vi "VI Main 1.21 - Copy.vi"() -> ()   [LabVIEW 2014]
uses:
  <vilib>/Analysis/baseanly.llb/Mean (DBL).vi
  <vilib>/Instr/_visa.llb/VISA Configure Serial Port (Instr).vi
  <vilib>/DAQmx/create/channels.llb/DAQmx Create Channel (AI-Voltage-Basic).vi
  <vilib>/DAQmx/configure/timing.llb/DAQmx Timing (Sample Clock).vi
  <vilib>/DAQmx/read.llb/DAQmx Read (Analog 2D DBL NChan NSamp).vi
  <vilib>/Utility/file.llb/Write To Spreadsheet File (DBL).vi
  <vilib>/Analysis/NI_AALPro.lvlib
  <vilib>/Analysis/NI_AALBase.lvlib
panel:
  out "T  (ºC)":dbl format="%.2g"
  out "RH  (%)":dbl format="%.2g"
  out "Ethanol (%)":dbl format="%.3g"
  out "MFC error IO":errorcluster={"status"=TRUE, "code"=0, "source"="VISA Read in MFC_Setpoint.vi->VI Main 1.21.vi"}
  out "KEITHLEY error IO":errorcluster={"status"=TRUE, "code"=0, "source"="Ke24xx Initialize.vi<ERR>Driver Status:  (Hex 0xBFFF0011) Insufficient location information or the device or resource is not present in the system."}
  out "DAQ error IO":errorcluster={"status"=TRUE, "code"=0, "source"="DAQmx Create Channel (AI-Voltage-Basic).vi:1780002<append>\n<B>Device Specified: </B>Dev2\n\n<B>Task Name: </B>_unnamedTask<29>"}
  out "Array 2":T1(array[cluster])=[{"ID"="-", "P(PSI)"=0.0, "T ºC"=0.0, "MassFlow"=0.0, "Setpoint"=0.0, "Gas"="-\r"}] {"Setpoint" format="%.2f"; "MassFlow" format="%.2f"}
  out "Linear?":bool=TRUE
  in  "Tab Control":enum32{"CONFIG", "Experiment"}(tab)=enum."Experiment"
  in  "resource RS232":string="ASRL4::INSTR"
  in  "resource GPIB":string="GPIB0::24::INSTR"
  out "status":i32=-1073807343 format="%.0x"
  in  "Reset":bool
  in  "COM:":bool=TRUE
  in  "RH/T Sensor VSS (V)":dbl=5.05 format="%.3g"
  in  "DAQ channels":tag="Dev1/ai21:23"
  in  "Rate (Hz)":dbl=1000.0
  in  "samples/channel":i32=100
  in  "K0":dbl=0.9054 format="%#_13g"
  in  "K1":dbl=-2.995 format="%#_13g"
  in  "Offset":dbl step=0.01 format="%_3f"
  in  "Gain":dbl=1.0
  in  "VISA COM Port":refnum<visa-resource-name>="COM3"
  in  "baud rate (9600)":u32=19200
  in  "Device ID's":string[](array[string])=["A", "B"]
  in  "Tare Flow":bool
  in  "Tare absP":bool
  in  "Disable MFC":bool
  in  "set 2":bool
  in  "MFC set2":cluster{"String":string, "MFC set":dbl}[](array[cluster])=[{"String"="A", "MFC set"=900.0}, {"String"="B", "MFC set"=100.0}] {"MFC set" format="%.2f"}
  in  "Speed":i32(slide)=2
  in  "# of points to acquire":i32=50 min=1 max=2500 step=1
  in  "Start (V)":dbl step=1.0 format="%.4p"
  in  "Ranging":i32(slide)
  in  "Direction":i32(slide)
  in  "Source compliance (A)":dbl=0.01 format="%.4f"
  in  "Stop (V)":dbl=5.0 format="%.4f"
  in  "Sense range":i32(slide)
  in  "Interval (s)":dbl=1.0 min=1.0 step=1.0
  in  "# of Intervals":i32=60 min=2 step=1
  out "Benchmark (s)":dbl format="%.2g"
  out "Current Interval":i32
  in  "Linear Fit \nResidue Threshold":dbl=0.1 format="%.3g"
  in  "clear graph":bool
  in  "clear graph at start":bool=TRUE
  in  "set 1":bool
  out "None linear \nIntervals":dbl[](array[numeric])
  in  "MFC set1":cluster{"String":string, "MFC set":dbl}[](array[cluster])=[{"String"="A", "MFC set"=1000.0}, {"String"="B", "MFC set"=100.0}] {"MFC set" format="%.2f"}
  in  "IV file path":path
  in  "Save IV to File":bool
  out "Start time":timestamp=timestamp(3638365108.305079 s since 1904-01-01)
  out "Elapsed Time":dbl format="%<%H:%M:%S>t"
  out "residue":dbl format="%#_3g"
  out "Measuring!":bool
  in  "STOP acq":bool
  in  "Quick Acq":bool
  in  "Multi Acq":bool
  in  "Single Acq":bool
  in  "stop":bool
  out "intercept":dbl format="%_4g"
  out "Waveform Chart":T2(graph)={"residue"=0.0, "residue"=0.0, "residue"=0.0, "residue"=0.0, "residue"=883.5, "residue"=0.0}
  out "Res. (ohm)":dbl format="%#.5g"
  out "XY Graph":cluster{dbl[], "Best Linear Fit":dbl[]}[](graph)
  out "Qrun":bool
  out "Mrun":bool
  out "Srun":bool
  # "Ethanol Sensor"
  # "RH%/T Sensor"
  # "MFC's"
  # "KEITHLEY"
  # ">"
  # "by L.Andrzejewski\nlandrzej@uottawa.ca"
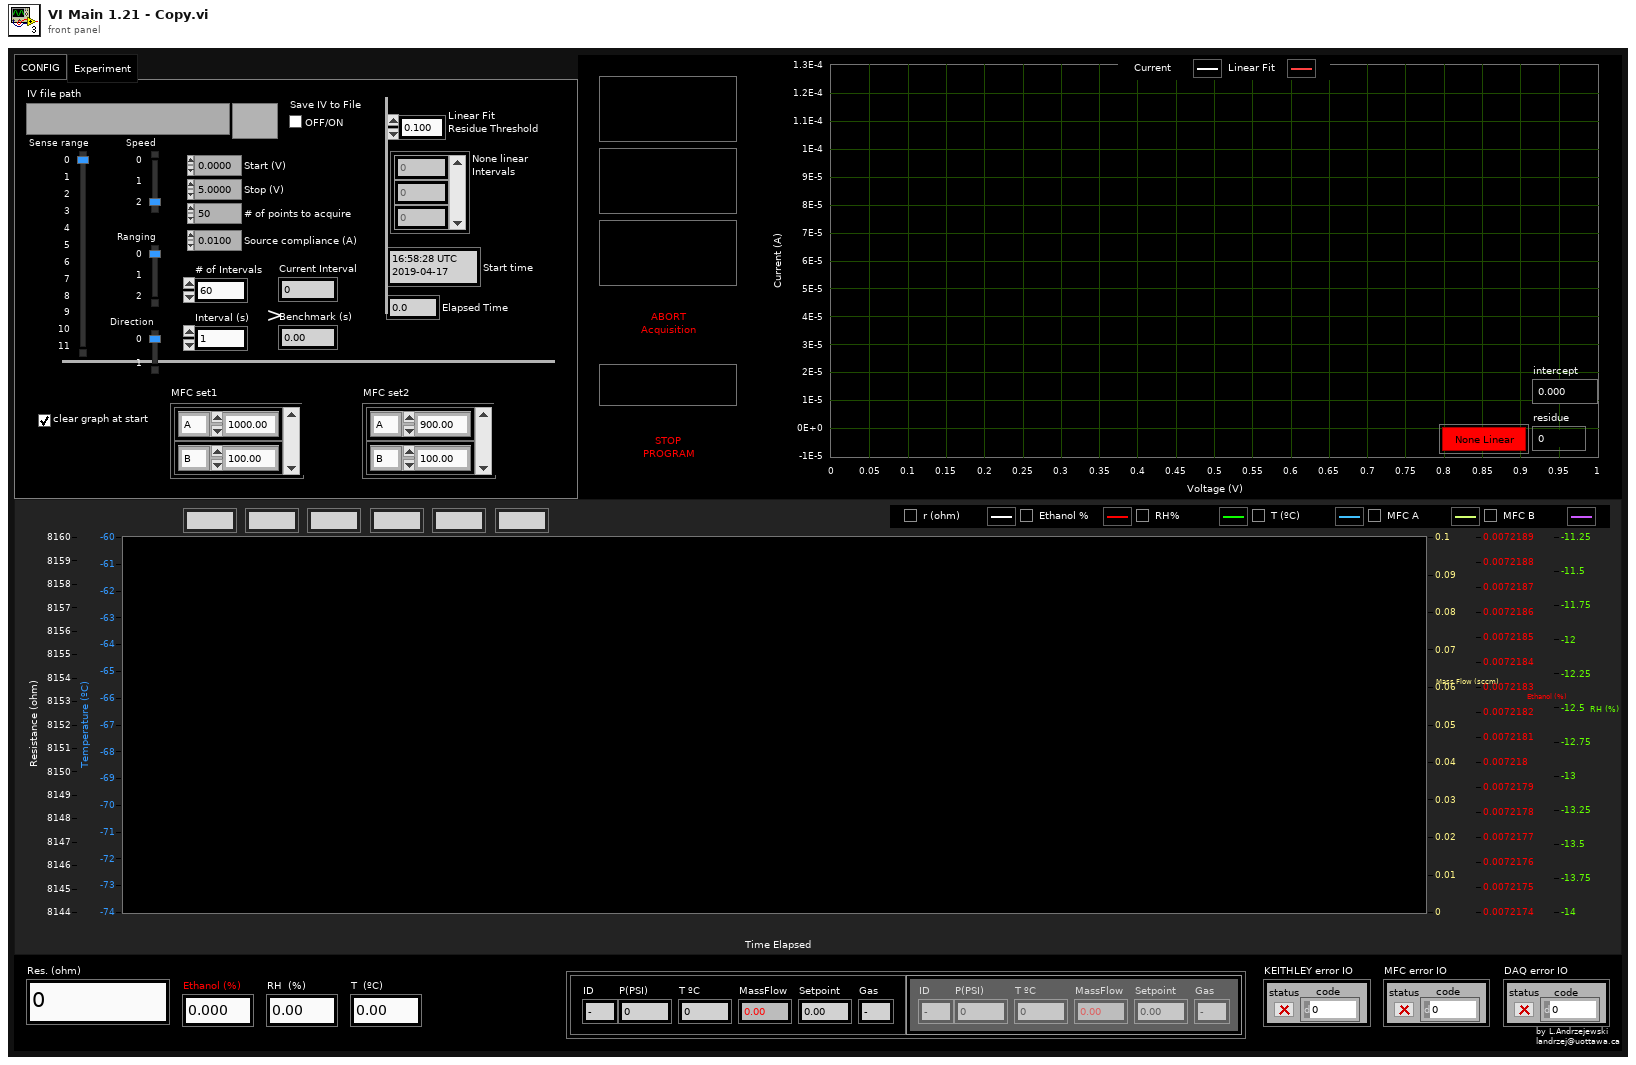
[diagram p1: front panel]
types:
  T1 = cluster{"ID":string, "P(PSI)":dbl, "T ºC":dbl, "MassFlow":dbl, "Setpoint":dbl, "Gas":string}[]
  T2 = cluster{"residue":dbl, "residue":dbl, "residue":dbl, "residue":dbl, "residue":dbl, "residue":dbl}
  T3 = enum8{"Enabled", "Disabled", "Disabled and Grayed Out"}
  T4 = cluster{"residue":dbl, "residue":dbl, "residue":dbl, "residue":dbl, "residue":dbl, "residue":dbl}[]
  T5 = cluster{dbl, dbl, dbl, dbl, "residue":dbl, "residue":dbl}
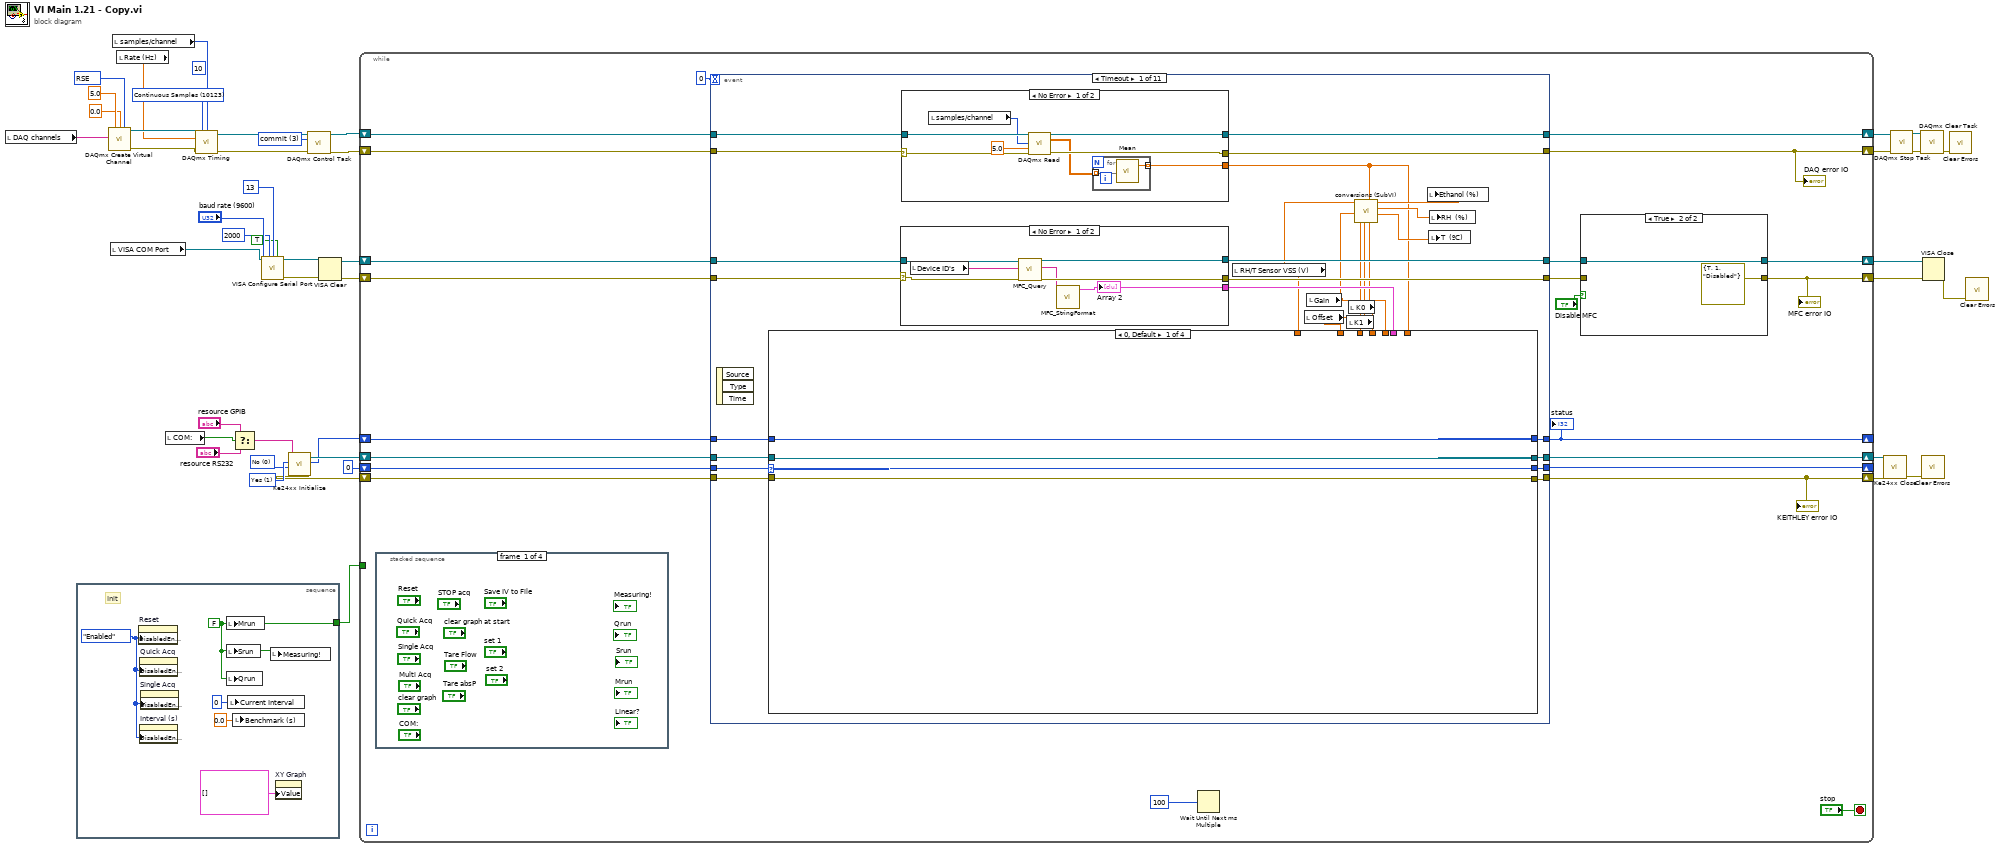
[diagram p0: block diagram]
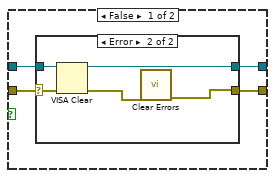
[diagram p2: hidden frame]
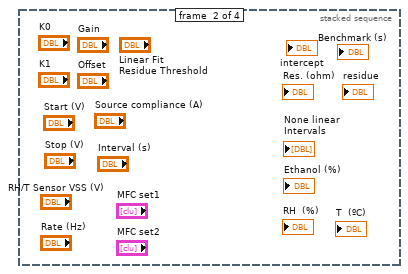
[diagram p4: hidden frame]
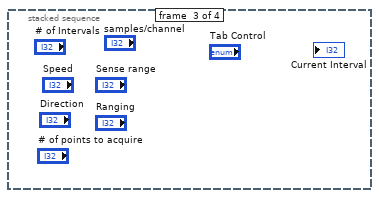
[diagram p5: hidden frame]
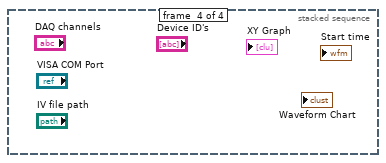
[diagram p6: hidden frame]
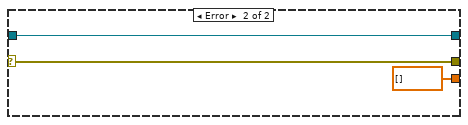
[diagram p7: hidden frame]
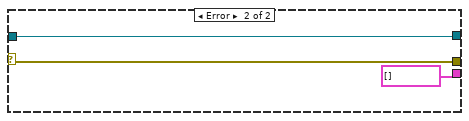
[diagram p8: hidden frame]
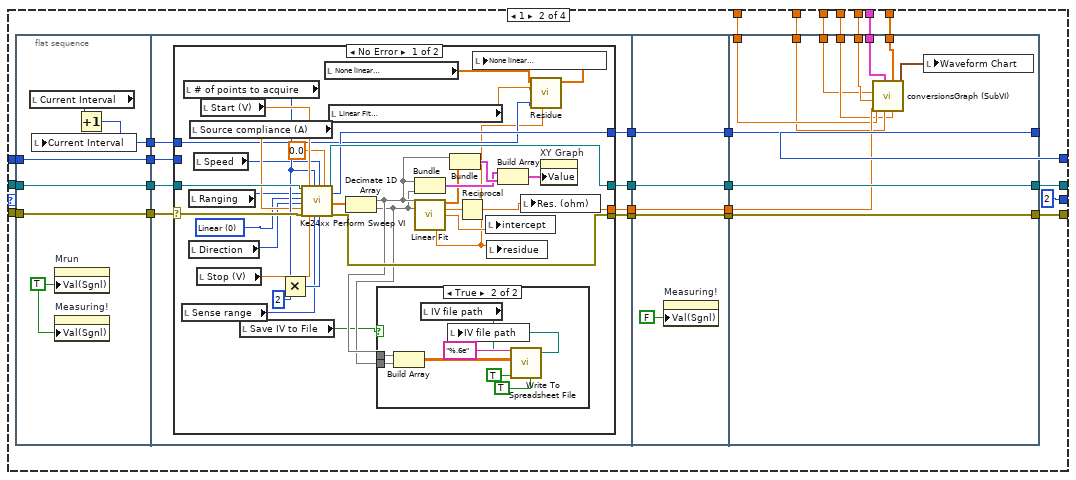
[diagram p9: hidden frame]
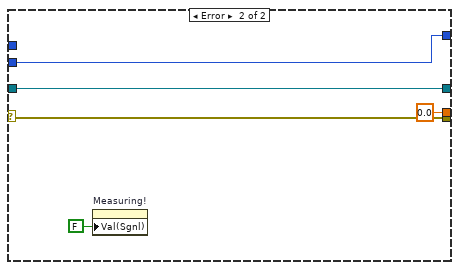
[diagram p11: hidden frame]
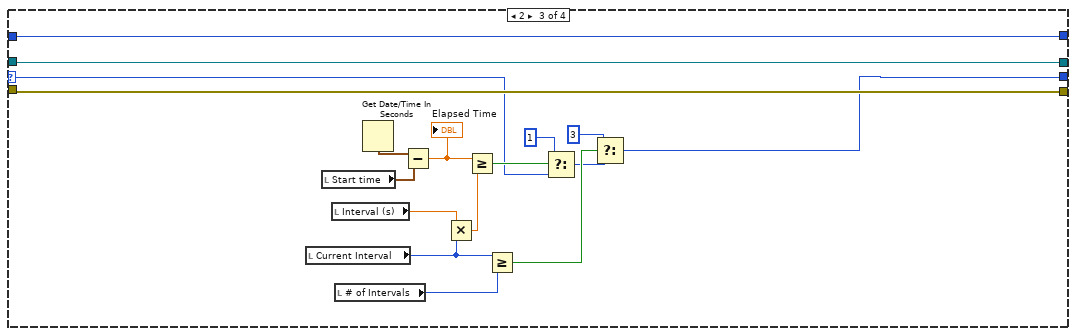
[diagram p12: hidden frame]
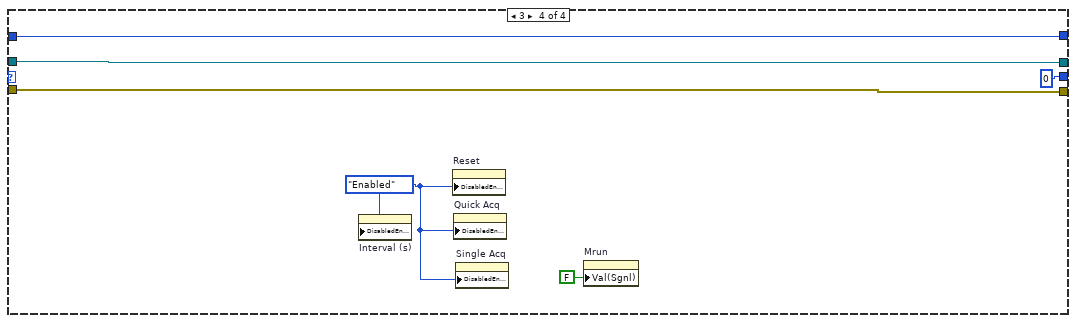
[diagram p13: hidden frame]
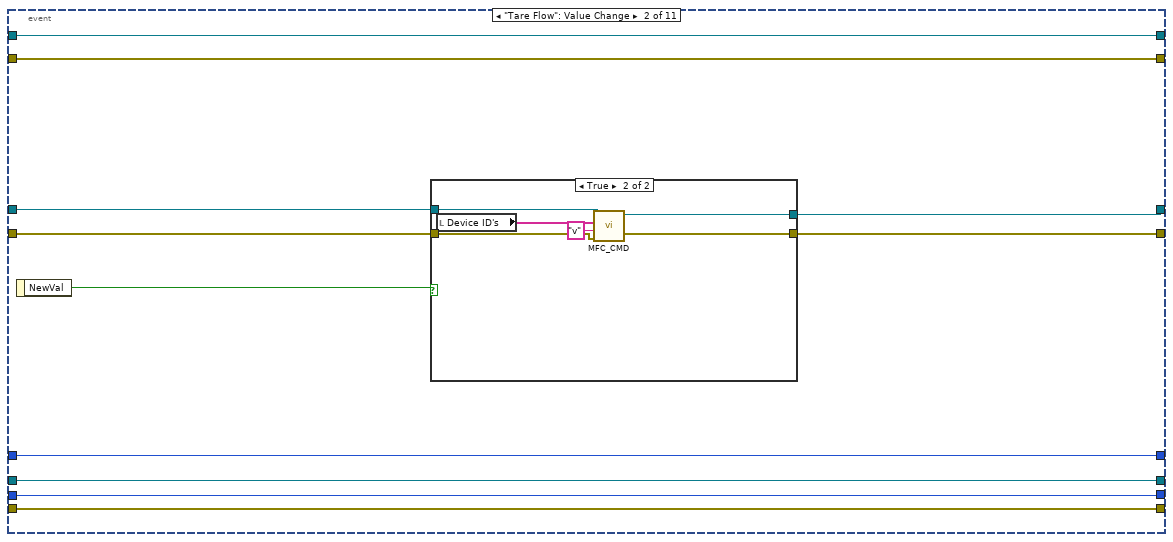
[diagram p14: hidden frame]
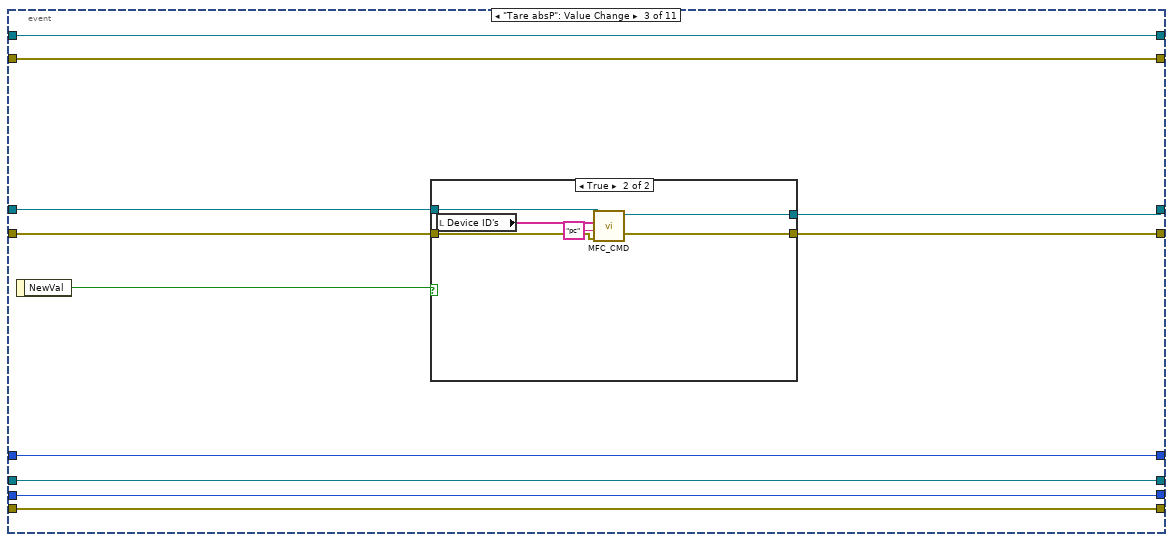
[diagram p16: hidden frame]
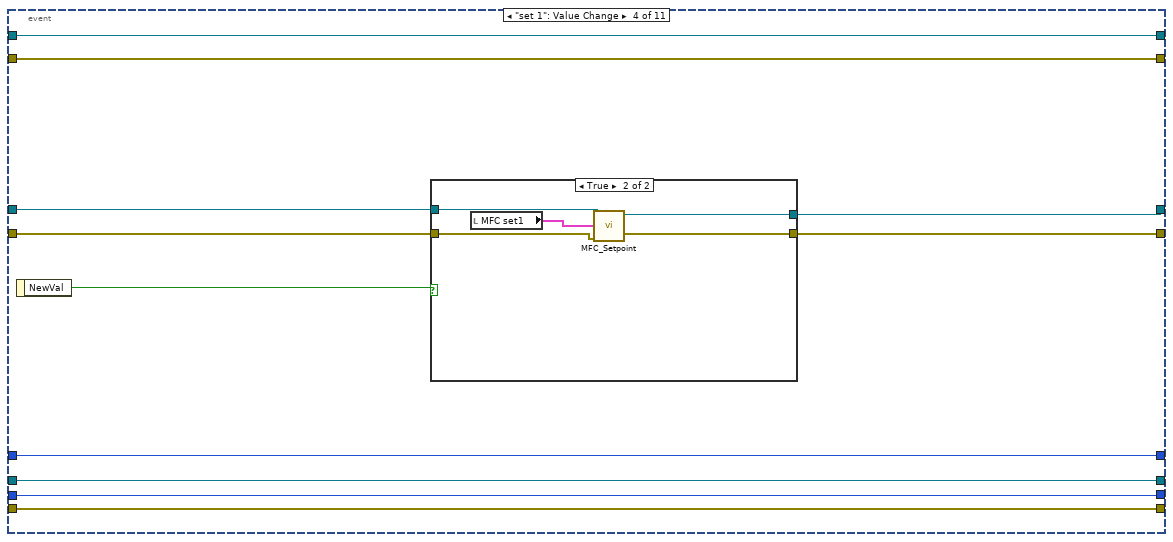
[diagram p18: hidden frame]
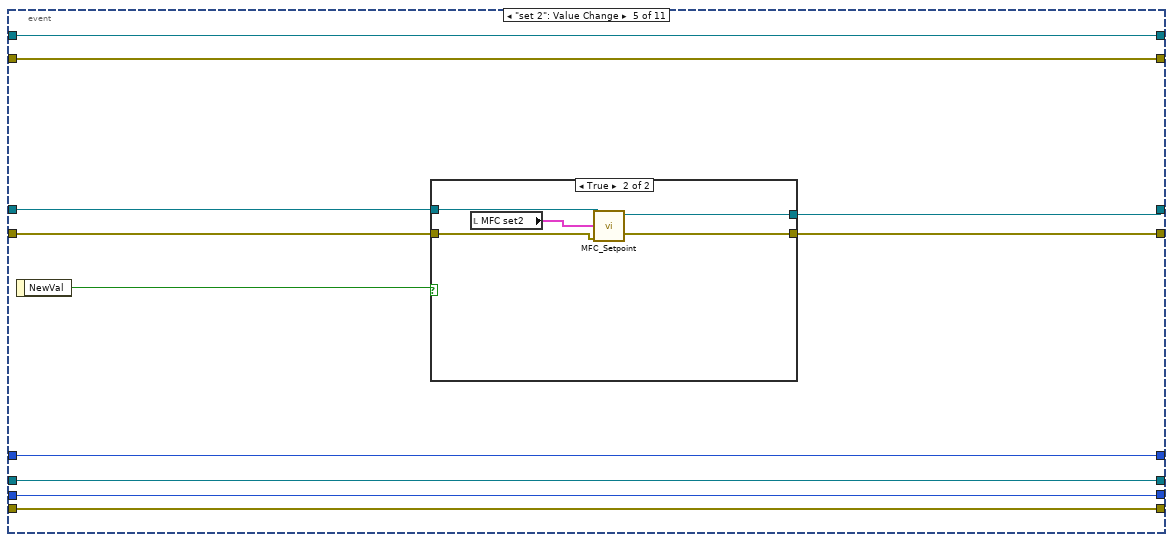
[diagram p20: hidden frame]
diagram:
  (unwired) 10 ("y")
  w3 = 3 items=["verify"=2, "reserve"=4, "commit"=3, "unreserve"=5, "abort"=6] ("action")
  w15 = 10123 items=["Finite Samples"=10178, "Continuous Samples"=10123, "Hardware Timed Single Point"=12522] ("sample mode")
  w17 = 10083 items=["default"=-1, "RSE"=10083, "NRSE"=10078, "Differential"=10106, "Pseudodifferential"=12529] ("input terminal configuration")
  w45 = u16 1 items=["Yes"=1, "No"=0] ("id query")
  w37 = u16 0 items=["Yes"=1, "No"=0] ("reset device")
  n1 = local read "DAQ channels"() -> (w12:tag)
  n2 = stacked-sequence {
    tunnel: [w48] -> w39
    frame #0 {
      w47 = T3."Enabled" ("Disabled")
      w48 = FALSE ("Mrun")
      # "Init"
      n3 = property on="Reset" class="Bool"("DisabledEnum"=w47) -> ()  [unwired: 2 in, 2 out]
      n4 = property on="Quick Acq" class="Bool"("DisabledEnum"=w47) -> ()  [unwired: 2 in, 2 out]
      n5 = property on="Interval (s)" class="DigNum (strict)"("DisabledEnum"=w47) -> ()  [unwired: 2 in, 2 out]
      n6 = property on="Single Acq" class="Bool"("DisabledEnum"=w47) -> ()  [unwired: 2 in, 2 out]
      n7 = local write "Mrun"(w48) -> ()
      n8 = local write "Srun"(w48) -> ()
      n9 = local write "Qrun"(w48) -> ()
      n10 = local write "Current Interval"(0 ("Current Interval")) -> ()
      n11 = local write "Benchmark (s)"(0.0 ("Benchmark (s)")) -> ()
      n12 = local write "Measuring!"(w48) -> ()
      n13 = property on="XY Graph" class="XYGraph (strict)"("Value"=cluster{dbl[], "Best Linear Fit":dbl[]}[] [] ("XY Graph")) -> ()  [unwired: 2 in, 2 out]
    }
  }
  n14 = call-poly <vilib>:"DAQmx Create Virtual Channel.vi"("maximum value"=5.0, "minimum value"=0.0, "input terminal configuration"=w17, "physical channels"=w12) -> ("task out"=w16:refnum<k21>, "error out"=w14:errorcluster)  [unwired: 10 in]
  n15 = local read "VISA COM Port"() -> (w20:refnum<visa-resource-name>)
  n16 = local read "samples/channel"() -> (w2:i32)
  n17 = local read "Rate (Hz)"() -> (w13:dbl)
  n18 = local read "COM:"() -> (w36:bool)
  n19 = call-poly <vilib>:"DAQmx Timing.vi"("task/channels in"=w16, "sample mode"=w15, "samples per channel"=w2, "rate"=w13, "error in"=w14) -> ("task out"=w1:refnum<k21>, "error out"=w4:errorcluster)  [unwired: 9 in]
  n20 = Select(t="resource GPIB", s=w36, f="resource RS232") -> (s? t:f=w33:string)
  n21 = call-poly "VISA Configure Serial Port"("VISA resource name"=w20, "timeout (10sec)"=u32 2000, "termination char\n(0xA = '\\n' = LF)"=u8 13 ("termination char\n(0xA = '\\n' = LF)"), "Enable Termination\nChar (T)"=TRUE ("Enable Termination\nChar (T)"), "baud rate (9600)"="baud rate (9600)") -> ("VISA resource name out"=w22:refnum<visa-resource-name>, "error out"=w21:errorcluster)  [unwired: 9 in]
  n22 = call "Ke24xx Initialize.vi"("reset device"=w37, "id query"=w45, "resource name"=w33) -> ("error out"=w40:errorcluster, "status"=w41:i32, "instrument handle out"=w42:refnum<visa-resource-name>)  [unwired: 6 in]
  n23 = call <vilib>:"DAQmx Control Task.vi"("task/channels in"=w1, "action"=w3, "error in"=w4) -> ("task out"=w6:refnum<k21>, "error out"=w5:errorcluster)  [unwired: 11 in]
  n24 = VISA Clear(VISA resource name=w22, error in (no error)=w21) -> (VISA resource name out=w24:refnum<visa-resource-name>, error out=w23:errorcluster)
  n25 = while {
    shift-right: [w67] -> w44
    shift-left: w42 -> [w69]
    shift-right: [w60] -> w43
    shift-left: w40 -> [w68]
    shift-right: [w65] -> _
    shift-left: w41 -> [w66]
    tunnel: w39 -> [_]
    shift-right: [w63] -> _
    shift-left: 0 -> [w64]
    shift-right: [w53] -> w28
    shift-left: w24 -> [w62]
    shift-right: [w55] -> w27
    shift-left: w23 -> [w61]
    shift-right: [w57] -> w9
    shift-left: w6 -> [w59]
    shift-right: [w52] -> w8
    shift-left: w5 -> [w58]
    stop <- "stop" stop-if-true
    n26 = stacked-sequence {
      frame #0 {
      }
      frame #1 {
      }
      frame #2 {
      }
      frame #3 {
      }
    }
    n27 = event shown="[0] Timeout" {
      selector: _ -> [_ _ _ _ _ _ _ _ _ _ _]
      dyn-events: _ -> [_ _ _ _ _ _ _ _ _ _ _]
      timeout: 0 -> [_ _ _ _ _ _ _ _ _ _ _]
      tunnel: [w107 w275 w294 w313 w331 w351 w376 w387 w462 w518 w537] -> w67
      tunnel: w69 -> [w110 w275 w294 w313 w331 w351 w376 w390 w465 w519 w537]
      tunnel: [w106 w273 w292 w311 w329 w350 w375 w388 w463 w517 w535] -> w60
      tunnel: w68 -> [w109 w273 w292 w311 w329 w350 w375 w389 w464 w516 w535]
      tunnel: w66 -> [w108 w272 w291 w310 w328 w347 w372 w386 w461 w521 w538]
      tunnel: [w104 w272 w291 w310 w328 w347 w372 w385 w460 w520 w538] -> w65
      tunnel: w64 -> [w111 w274 w293 w312 w330 w348 w373 w384 w459 w515 w536]
      tunnel: [w105 w274 w293 w312 w330 w349 w374 w384 w459 w515 w536] -> w63
      tunnel: [w102 w268 w287 w306 w324 w345 w370 w382 w457 w513 w533] -> w54
      tunnel: w62 -> [w97 w270 w289 w308 w326 w345 w370 w382 w457 w513 w533]
      tunnel: [w103 w267 w286 w305 w323 w346 w371 w383 w458 w514 w534] -> w56
      tunnel: w61 -> [w96 w269 w288 w307 w325 w346 w371 w383 w458 w514 w534]
      tunnel: [w99 w266 w285 w304 w322 w344 w369 w381 w456 w512 w532] -> w57
      tunnel: w59 -> [w86 w266 w285 w304 w322 w344 w369 w381 w456 w512 w532]
      tunnel: [w98 w265 w284 w303 w321 w343 w368 w380 w455 w511 w531] -> w52
      tunnel: w58 -> [w100 w265 w284 w303 w321 w343 w368 w380 w455 w511 w531]
      event Timeout {
        n28 = event-data() -> ()  [unwired: 1 in, 3 out]
        n29 = case shown="No Error" w96 {
          selector: w96 -> [w129 w133]
          tunnel: w97 -> [w130 w134]
          tunnel: [w128 w133] -> w103
          tunnel: [w127 w134] -> w102
          tunnel: [w125 T1 [] ("Array out")] -> w101
          frame No Error {
            n30 = local read "Device ID's"() -> (w131:string[])
            n31 = call "MFC_Query.vi"("error in (no error)"=w129, "Device ID's"=w131, "VISA Refnum in"=w130) -> ("error out"=w128:errorcluster, "Array"=w126:string[], "VISA Refnum out"=w127:refnum<visa-resource-name>)  [unwired: 6 in]
            n32 = call "MFC_StringFormat.vi"("Array"=w126) -> ("Array out"=w125:T1)  [unwired: 10 in]
            "Array 2" <- w125
          }
          frame Error {
          }
        }
        n33 = case shown="No Error" w100 {
          selector: w100 -> [w115 w123]
          tunnel: [w118 w124] -> w99
          tunnel: w86 -> [w119 w124]
          tunnel: [w114 w123] -> w98
          tunnel: [w112 dbl[] []] -> w92
          frame No Error {
            n34 = local read "samples/channel"() -> (w116:i32)
            n35 = call-poly <vilib>:"DAQmx Read.vi"("task/channels in"=w119, "number of samples per channel"=w116, "timeout"=5.0, "error in"=w115) -> ("task out"=w118:refnum<k21>, "data"=w113:dbl[][], "error out"=w114:errorcluster)  [unwired: 9 in]
            n36 = for {
              tunnel: w113 -> [w121] mode=indexing
              tunnel: [w120] -> w112 mode=indexing
              n37 = call-poly <vilib>:"Mean.vi"("X"=w121) -> ("mean"=w120:dbl)  [unwired: 1 out]
            }
          }
          frame Error {
          }
        }
        n38 = local read "RH/T Sensor VSS (V)"() -> (w91:dbl)
        n39 = local read "Offset"() -> (w88:dbl)
        n40 = local read "Gain"() -> (w89:dbl)
        n41 = local read "K1"() -> (w90:dbl)
        n42 = local read "K0"() -> (w87:dbl)
        n43 = case shown="0, Default" w111 {
          selector: w111 -> [w135 _ w247 _]
          tunnel: w110 -> [w137 w162 w256 w262]
          tunnel: w109 -> [w136 w161 w257 w260]
          tunnel: w108 -> [w138 w145 w258 w263]
          tunnel: [w137 w160 w256 w262] -> w107
          tunnel: [w136 w159 w257 w260] -> w106
          tunnel: [w135 2 w244 0 ("t")] -> w105
          tunnel: [w138 w157 w258 w263] -> w104
          tunnel: w101 -> [_ w150 _ _]
          tunnel: w92 -> [_ w149 _ _]
          tunnel: w91 -> [_ w143 _ _]
          tunnel: w89 -> [_ w142 _ _]
          tunnel: w88 -> [_ w141 _ _]
          tunnel: w87 -> [_ w140 _ _]
          tunnel: w90 -> [_ w139 _ _]
          frame 0, Default {
          }
          frame 1 {
            n44 = flat-sequence {
              tunnel: w161 -> [w169]
              tunnel: w162 -> [w170]
              tunnel: [w170] -> w164
              tunnel: [w169] -> w163
              tunnel: [w167] -> w146
              tunnel: w145 -> [w167]
              tunnel: [w165] -> w144
              tunnel: w164 -> [w178]
              tunnel: w163 -> [w177]
              tunnel: [w176] -> w156
              tunnel: [w175] -> w155
              tunnel: [w174] -> w154
              tunnel: [w173] -> w147
              tunnel: w146 -> [w172]
              tunnel: w144 -> [w171]
              tunnel: w156 -> [w229]
              tunnel: w155 -> [w228]
              tunnel: w154 -> [w227]
              tunnel: [w229] -> w153
              tunnel: [w228] -> w152
              tunnel: [w227] -> w151
              tunnel: [w225] -> w148
              tunnel: w147 -> [w225]
              tunnel: [w239] -> w157
              tunnel: [w240] -> w160
              tunnel: [w241] -> w159
              tunnel: w153 -> [w241]
              tunnel: w152 -> [w240]
              tunnel: w151 -> [w239]
              tunnel: w150 -> [w235]
              tunnel: w149 -> [w236]
              tunnel: w148 -> [w237]
              tunnel: w143 -> [w234]
              tunnel: w142 -> [w233]
              tunnel: w141 -> [w232]
              tunnel: w140 -> [w231]
              tunnel: w139 -> [w230]
              frame #0 {
                w166 = TRUE ("Value (Signaling)")
                n45 = local read "Current Interval"() -> (w168:i32)
                n46 = property on="Mrun" class="Bool (strict)"("Val(Sgnl)"=w166) -> ()  [unwired: 2 in, 2 out]
                n47 = property on="Measuring!" class="Bool (strict)"("Val(Sgnl)"=w166) -> ()  [unwired: 2 in, 2 out]
                n48 = Increment(x=w168) -> (x+1=w165:i32)
                n49 = local write "Current Interval"(w165) -> ()
              }
              frame #1 {
                n50 = case shown="No Error" w177 {
                  selector: w177 -> [w205 w223]
                  tunnel: w178 -> [w206 w224]
                  tunnel: [w204 w223] -> w176
                  tunnel: [w203 w224] -> w175
                  tunnel: [w188 w221] -> w174
                  tunnel: [w187 0.0] -> w173
                  tunnel: w172 -> [_ w221]
                  tunnel: w171 -> [w181 _]
                  frame No Error {
                    w190 = 0 items=["Linear", "Logarithmic"] ("spacing")
                    n51 = local read "Sense range"() -> (w195:i32)
                    n52 = local read "# of points to acquire"() -> (w197:i32)
                    n53 = local read "Ranging"() -> (w192:i32)
                    n54 = local read "Direction"() -> (w191:i32)
                    n55 = local read "Source compliance (A)"() -> (w194:dbl)
                    n56 = local read "Speed"() -> (w193:i32)
                    n57 = local read "Stop (V)"() -> (w199:dbl)
                    n58 = local read "Start (V)"() -> (w200:dbl)
                    n59 = local read "Save IV to File"() -> (w184:bool)
                    n60 = Multiply(x=w197, y=2) -> (x*y=w196:i32)
                    n61 = call "Ke24xx Perform Sweep VI.vi"("instrument handle"=w206, "ranging"=w192, "spacing"=w190, "direction"=w191, "source compliance"=w194, "error in (no error)"=w205, "start"=w200, "stop"=w199, "number of points"=w197, "sense range"=w195, "speed"=w193, "size of reading"=w196, "source protection"=0.0) -> ("instrument handle out"=w203:refnum<visa-resource-name>, "status"=w188:i32, "out"=w207:dbl[], "error out"=w204:errorcluster)  [unwired: 3 in]
                    n62 = local read "None linear \nIntervals"() -> (w183:dbl[])
                    n63 = local read "Linear Fit \nResidue Threshold"() -> (w180:dbl)
                    n64 = Decimate 1D Array(w207) -> (w186:dbl[], w185:dbl[])
                    n65 = case shown="True" w184 {
                      tunnel: w186 -> [_ w219]
                      tunnel: w185 -> [_ w218]
                      frame False {
                      }
                      frame True {
                        n66 = Build Array(w219, w218) -> (w214:dbl[][])
                        n67 = local read "IV file path"() -> (w215:path)
                        n68 = call-poly <vilib>:"Write To Spreadsheet File.vi"("transpose? (no:F)"=TRUE, "format (%.3f)"="%.6e", "append to file? (new file:F)"=TRUE, "2D data"=w214, "file path (dialog if empty)"=w215) -> ("new file path (Not A Path if cancelled)"=w213:path)  [unwired: 3 in]
                        n69 = local write "IV file path"(w213) -> ()
                      }
                    }
                    n70 = Bundle(w186, w185) -> (w210:cluster{dbl[], dbl[]})  [unwired: 1 in]
                    n71 = call <vilib>:"Linear Fit.vi"("Y"=w185, "X"=w186) -> ("Best Linear Fit"=w209:dbl[], "slope"=w208:dbl, "intercept"=w202:dbl, "residue"=w179:dbl)  [unwired: 9 in, 1 out]
                    n72 = Bundle(w186, "Best Linear Fit"=w209) -> (w211:cluster{dbl[], "Best Linear Fit":dbl[]})  [unwired: 1 in]
                    n73 = Reciprocal(x=w208) -> (1/x=w187:dbl)
                    n74 = local write "intercept"(w202) -> ()
                    n75 = local write "residue"(w179) -> ()
                    n76 = Build Array(w210, w211) -> (w201:cluster{dbl[], "Best Linear Fit":dbl[]}[])
                    n77 = local write "Res. (ohm)"(w187) -> ()
                    n78 = call "Residue.vi"("residue"=w179, "Current Interval"=w181, "Linear Fit \nResidue Threshold"=w180, "None linear \nIntervals IN"=w183) -> ("None linear \nIntervals OUT"=w182:dbl[])  [unwired: 7 in]
                    n79 = local write "None linear \nIntervals"(w182) -> ()
                    n80 = property on="XY Graph" class="XYGraph (strict)"("Value"=w201) -> ()  [unwired: 2 in, 2 out]
                  }
                  frame Error {
                    n81 = property on="Measuring!" class="Bool (strict)"("Val(Sgnl)"=FALSE ("Value (Signaling)")) -> ()  [unwired: 2 in, 2 out]
                  }
                }
              }
              frame #2 {
                n82 = property on="Measuring!" class="Bool (strict)"("Val(Sgnl)"=FALSE ("Value (Signaling)")) -> ()  [unwired: 2 in, 2 out]
              }
              frame #3 {
                n83 = call "conversionsGraph (SubVI).vi"("K0"=w231, "Array"=w236, "Offset"=w232, "Array in"=w235, "Numeric"=w237, "Gain"=w233, "K1"=w230, "RH/T Sensor VSS (V)"=w234) -> ("Cluster"=w238:T5)  [unwired: 3 in]
                n84 = local write "Waveform Chart"(w238) -> ()
              }
            }
          }
          frame 2 {
            n85 = local read "Current Interval"() -> (w250:i32)
            n86 = local read "Start time"() -> (w254:timestamp)
            n87 = local read "Interval (s)"() -> (w253:dbl)
            n88 = local read "# of Intervals"() -> (w249:i32)
            n89 = Get Date/Time In Seconds() -> (seconds since 1Jan1904=w255:timestamp)
            n90 = Subtract(x=w255, y=w254) -> (x-y=w242:dbl)
            "Elapsed Time" <- w242
            n91 = Multiply(x=w253, y=w250) -> (x*y=w252:dbl)
            n92 = Greater Or Equal?(x=w242, y=w252) -> (x >= y?=w251:bool)
            n93 = Greater Or Equal?(x=w250, y=w249) -> (x >= y?=w246:bool)
            n94 = Select(t=1, s=w251, f=w247) -> (s? t:f=w245:i32)
            n95 = Select(t=3, s=w246, f=w245) -> (s? t:f=w244:i32)
          }
          frame 3 {
            w259 = T3."Enabled" ("Disabled")
            n96 = property on="Interval (s)" class="DigNum (strict)"("DisabledEnum"=w259) -> ()  [unwired: 2 in, 2 out]
            n97 = property on="Reset" class="Bool"("DisabledEnum"=w259) -> ()  [unwired: 2 in, 2 out]
            n98 = property on="Quick Acq" class="Bool"("DisabledEnum"=w259) -> ()  [unwired: 2 in, 2 out]
            n99 = property on="Single Acq" class="Bool"("DisabledEnum"=w259) -> ()  [unwired: 2 in, 2 out]
            n100 = property on="Mrun" class="Bool (strict)"("Val(Sgnl)"=FALSE ("Value (Signaling)")) -> ()  [unwired: 2 in, 2 out]
          }
        }
        n101 = call "conversions (SubVI).vi"("K0"=w87, "Array"=w92, "Offset"=w88, "Gain"=w89, "K1"=w90, "RH/T Sensor VSS (V)"=w91) -> ("T"=w93:dbl, "RH"=w94:dbl, "Ethanol"=w95:dbl)  [unwired: 3 in]
        n102 = local write "Ethanol (%)"(w95) -> ()
        n103 = local write "T  (ºC)"(w93) -> ()
        n104 = local write "RH  (%)"(w94) -> ()
      }
      event "Tare Flow": Value Change {
        n105 = event-data() -> ("NewVal"=w271:bool)  [unwired: 1 in]
        n106 = case shown="True" w271 {
          tunnel: w270 -> [w277 w283]
          tunnel: w269 -> [w276 w282]
          tunnel: [w277 w281] -> w268
          tunnel: [w276 w280] -> w267
          frame False {
          }
          frame True {
            n107 = local read "Device ID's"() -> (w279:string[])
            n108 = call "MFC_CMD.vi"("error in (no error)"=w282, "cmd"="v", "Device ID's"=w279, "VISA Refnum in"=w283) -> ("error out"=w280:errorcluster, "VISA Refnum out"=w281:refnum<visa-resource-name>)  [unwired: 6 in]
          }
        }
      }
      event "Tare absP": Value Change {
        n109 = event-data() -> ("NewVal"=w290:bool)  [unwired: 1 in]
        n110 = case shown="True" w290 {
          tunnel: w289 -> [w296 w302]
          tunnel: w288 -> [w295 w301]
          tunnel: [w296 w300] -> w287
          tunnel: [w295 w299] -> w286
          frame False {
          }
          frame True {
            n111 = local read "Device ID's"() -> (w298:string[])
            n112 = call "MFC_CMD.vi"("error in (no error)"=w301, "cmd"="pc", "Device ID's"=w298, "VISA Refnum in"=w302) -> ("error out"=w299:errorcluster, "VISA Refnum out"=w300:refnum<visa-resource-name>)  [unwired: 6 in]
          }
        }
      }
      event "set 1": Value Change {
        n113 = event-data() -> ("NewVal"=w309:bool)  [unwired: 1 in]
        n114 = case shown="True" w309 {
          tunnel: w308 -> [w315 w320]
          tunnel: w307 -> [w314 w319]
          tunnel: [w315 w318] -> w306
          tunnel: [w314 w317] -> w305
          frame False {
          }
          frame True {
            n115 = local read "MFC set1"() -> (w316:cluster{"String":string, "MFC set":dbl}[])
            n116 = call "MFC_Setpoint.vi"("error in (no error)"=w319, "MFC set1"=w316, "VISA Refnum in"=w320) -> ("error out"=w317:errorcluster, "VISA Refnum out"=w318:refnum<visa-resource-name>)  [unwired: 7 in]
          }
        }
      }
      event "set 2": Value Change {
        n117 = event-data() -> ("NewVal"=w327:bool)  [unwired: 1 in]
        n118 = case shown="True" w327 {
          tunnel: w326 -> [w333 w338]
          tunnel: w325 -> [w332 w337]
          tunnel: [w333 w336] -> w324
          tunnel: [w332 w335] -> w323
          frame False {
          }
          frame True {
            n119 = local read "MFC set2"() -> (w334:cluster{"String":string, "MFC set":dbl}[])
            n120 = call "MFC_Setpoint.vi"("error in (no error)"=w337, "MFC set1"=w334, "VISA Refnum in"=w338) -> ("error out"=w335:errorcluster, "VISA Refnum out"=w336:refnum<visa-resource-name>)  [unwired: 7 in]
          }
        }
      }
      event "Multi Acq": Value Change {
        n121 = event-data() -> ("NewVal"=w352:bool)  [unwired: 1 in]
        n122 = local read "IV file path"() -> (w339:path)
        n123 = local read "Save IV to File"() -> (w340:bool)
        n124 = Empty String/Path?(string/path=w339) -> (empty?=w342:bool)
        n125 = And(x=w342, y=w340) -> (x .and. y?=w341:bool)
        n126 = case shown="False" w341 {
          tunnel: w352 -> [w355 _]
          tunnel: [w354 0] -> w349
          tunnel: w348 -> [w353 _]
          frame False {
            n127 = case shown="True" w355 {
              tunnel: [w356 1] -> w354
              tunnel: w353 -> [w356 _]
              frame False {
              }
              frame True {
                w360 = T3."Disabled and Grayed Out" ("Disabled")
                n128 = local read "clear graph at start"() -> (w359:bool)
                n129 = Get Date/Time In Seconds() -> (seconds since 1Jan1904=w362:timestamp)
                n130 = local read "Interval (s)"() -> (w361:dbl)
                n131 = local write "Start time"(w362) -> ()
                n132 = property on="Interval (s)" class="DigNum (strict)"("DisabledEnum"=w360) -> ()  [unwired: 2 in, 2 out]
                n133 = local write "Current Interval"(0 ("Current Interval")) -> ()
                n134 = local write "None linear \nIntervals"(dbl[] [] ("None linear Intervals")) -> ()
                n135 = property on="Waveform Chart" class="WFChart (strict)"("XScale.Multiplier"=w361) -> ()  [unwired: 2 in, 2 out]
                n136 = case shown="True" w359 {
                  frame False {
                  }
                  frame True {
                    n137 = property on="Waveform Chart" class="WFChart (strict)"("History Data"=T4 []) -> ()  [unwired: 2 in, 2 out]
                  }
                }
                n138 = property on="Reset" class="Bool"("DisabledEnum"=w360) -> ()  [unwired: 2 in, 2 out]
                n139 = property on="Quick Acq" class="Bool"("DisabledEnum"=w360) -> ()  [unwired: 2 in, 2 out]
                n140 = property on="Single Acq" class="Bool"("DisabledEnum"=w360) -> ()  [unwired: 2 in, 2 out]
                n141 = property on="XY Graph" class="XYGraph (strict)"("Value"=cluster{dbl[], "Best Linear Fit":dbl[]}[] [] ("XY Graph")) -> ()  [unwired: 2 in, 2 out]
              }
            }
          }
          frame True {
            n142 = One Button Dialog(message="File path empty, Multi Acquisition Canceled") -> ()  [unwired: 1 in, 1 out]
          }
        }
      }
      event "STOP acq": Value Change {
        n143 = event-data() -> ("NewVal"=w377:bool)  [unwired: 1 in]
        n144 = case shown="True" w377 {
          tunnel: [w378 3] -> w374
          tunnel: w373 -> [w378 _]
          frame False {
          }
          frame True {
          }
        }
      }
      event "Single Acq": Value Change {
        n145 = event-data() -> ("NewVal"=w391:bool)  [unwired: 1 in]
        n146 = case shown="True" w391 {
          tunnel: w390 -> [w394 w409]
          tunnel: w389 -> [w393 w408]
          tunnel: [w393 w407] -> w388
          tunnel: [w394 w406] -> w387
          tunnel: [w392 w401] -> w385
          tunnel: w386 -> [w392 _]
          frame False {
          }
          frame True {
            n147 = flat-sequence {
              tunnel: w408 -> [w412]
              tunnel: w409 -> [w413]
              tunnel: [w413] -> w403
              tunnel: [w412] -> w402
              tunnel: [w410] -> w398
              tunnel: [w434] -> w405
              tunnel: [w433] -> w404
              tunnel: w403 -> [w436]
              tunnel: w402 -> [w435]
              tunnel: [w417] -> w400
              tunnel: [w453] -> w406
              tunnel: [w454] -> w407
              tunnel: w405 -> [w454]
              tunnel: w404 -> [w453]
              tunnel: [w452] -> w401
              tunnel: w400 -> [w452]
              tunnel: [w450] -> w399
              frame #0 {
                n148 = Tick Count (ms)() -> (millisecond timer value=w410:u32)
                n149 = property on="Srun" class="Bool (strict)"("Val(Sgnl)"=TRUE ("Value (Signaling)")) -> ()  [unwired: 2 in, 2 out]
              }
              frame #1 {
                w419 = 0 items=["Linear", "Logarithmic"] ("spacing")
                n150 = local read "# of points to acquire"() -> (w426:i32)
                n151 = local read "Ranging"() -> (w421:i32)
                n152 = local read "Direction"() -> (w420:i32)
                n153 = local read "Source compliance (A)"() -> (w423:dbl)
                n154 = local read "Speed"() -> (w422:i32)
                n155 = local read "Stop (V)"() -> (w428:dbl)
                n156 = local read "Start (V)"() -> (w429:dbl)
                n157 = local read "Sense range"() -> (w424:i32)
                n158 = local read "Save IV to File"() -> (w416:bool)
                n159 = Multiply(x=w426, y=2) -> (x*y=w425:i32)
                n160 = call "Ke24xx Perform Sweep VI.vi"("instrument handle"=w436, "ranging"=w421, "spacing"=w419, "direction"=w420, "source compliance"=w423, "error in (no error)"=w435, "start"=w429, "stop"=w428, "number of points"=w426, "sense range"=w424, "speed"=w422, "size of reading"=w425, "source protection"=0.0) -> ("instrument handle out"=w433:refnum<visa-resource-name>, "status"=w417:i32, "out"=w437:dbl[], "error out"=w434:errorcluster)  [unwired: 3 in]
                n161 = Decimate 1D Array(w437) -> (w415:dbl[], w414:dbl[])
                n162 = case shown="True" w416 {
                  tunnel: w415 -> [_ w449]
                  tunnel: w414 -> [_ w448]
                  frame False {
                  }
                  frame True {
                    n163 = Build Array(w449, w448) -> (w444:dbl[][])
                    n164 = local read "IV file path"() -> (w445:path)
                    n165 = call-poly <vilib>:"Write To Spreadsheet File.vi"("transpose? (no:F)"=TRUE, "format (%.3f)"="%.6e", "append to file? (new file:F)"=TRUE, "2D data"=w444, "file path (dialog if empty)"=w445) -> ("new file path (Not A Path if cancelled)"=w443:path)  [unwired: 3 in]
                    n166 = local write "IV file path"(w443) -> ()
                  }
                }
                n167 = Bundle(w415, w414) -> (w440:cluster{dbl[], dbl[]})  [unwired: 1 in]
                n168 = call <vilib>:"Linear Fit.vi"("Y"=w414, "X"=w415) -> ("Best Linear Fit"=w439:dbl[], "slope"=w438:dbl, "intercept"=w432:dbl)  [unwired: 9 in, 2 out]
                n169 = Bundle(w415, "Best Linear Fit"=w439) -> (w441:cluster{dbl[], "Best Linear Fit":dbl[]})  [unwired: 1 in]
                n170 = Reciprocal(x=w438) -> (1/x=w431:dbl)
                n171 = local write "intercept"(w432) -> ()
                n172 = Build Array(w440, w441) -> (w430:cluster{dbl[], "Best Linear Fit":dbl[]}[])
                n173 = local write "Res. (ohm)"(w431) -> ()
                n174 = property on="XY Graph" class="XYGraph (strict)"("Value"=w430) -> ()  [unwired: 2 in, 2 out]
              }
              frame #2 {
                n175 = Tick Count (ms)() -> (millisecond timer value=w450:u32)
                n176 = property on="Srun" class="Bool (strict)"("Val(Sgnl)"=FALSE ("Value (Signaling)")) -> ()  [unwired: 2 in, 2 out]
              }
            }
            n177 = Subtract(x=w399, y=w398) -> (x-y=w397:u32)
            n178 = Divide(x=w397, y=u32 1000) -> (x/y=w395:dbl)
            n179 = local write "Benchmark (s)"(w395) -> ()
          }
        }
      }
      event "Quick Acq": Value Change {
        n180 = event-data() -> ("NewVal"=w466:bool)  [unwired: 1 in]
        n181 = case shown="True" w466 {
          tunnel: w465 -> [w469 w479]
          tunnel: w464 -> [w468 w478]
          tunnel: [w468 w477] -> w463
          tunnel: [w469 w476] -> w462
          tunnel: [w467 w471] -> w460
          tunnel: w461 -> [w467 _]
          frame False {
          }
          frame True {
            n182 = flat-sequence {
              tunnel: w478 -> [w481]
              tunnel: w479 -> [w482]
              tunnel: [w482] -> w475
              tunnel: [w481] -> w474
              tunnel: w475 -> [w502]
              tunnel: w474 -> [w501]
              tunnel: [w500] -> w473
              tunnel: [w499] -> w472
              tunnel: [w485] -> w470
              tunnel: [w509] -> w476
              tunnel: [w510] -> w477
              tunnel: w473 -> [w510]
              tunnel: w472 -> [w509]
              tunnel: [w507] -> w471
              tunnel: w470 -> [w507]
              frame #0 {
                n183 = property on="Qrun" class="Bool (strict)"("Val(Sgnl)"=TRUE ("Qrun")) -> ()  [unwired: 2 in, 2 out]
              }
              frame #1 {
                w486 = 2 items=["Slow", "Medium", "Fast"] ("speed")
                w487 = 2 ("x")
                w489 = 0 items=["Linear", "Logarithmic"] ("spacing")
                n184 = local read "Ranging"() -> (w491:i32)
                n185 = local read "Direction"() -> (w490:i32)
                n186 = local read "Source compliance (A)"() -> (w492:dbl)
                n187 = local read "Stop (V)"() -> (w496:dbl)
                n188 = local read "Start (V)"() -> (w497:dbl)
                n189 = local read "Sense range"() -> (w493:i32)
                n190 = Multiply(x=w487, y=2) -> (x*y=w494:i32)
                n191 = call "Ke24xx Perform Sweep VI.vi"("instrument handle"=w502, "ranging"=w491, "spacing"=w489, "direction"=w490, "source compliance"=w492, "error in (no error)"=w501, "start"=w497, "stop"=w496, "number of points"=w487, "sense range"=w493, "speed"=w486, "size of reading"=w494, "source protection"=0.0) -> ("instrument handle out"=w499:refnum<visa-resource-name>, "status"=w485:i32, "out"=w503:dbl[], "error out"=w500:errorcluster)  [unwired: 3 in]
                n192 = Decimate 1D Array(w503) -> (w506:dbl[], w504:dbl[])
                n193 = call <vilib>:"Linear Fit.vi"("Y"=w504, "X"=w506) -> ("slope"=w505:dbl, "intercept"=w498:dbl, "residue"=w483:dbl)  [unwired: 9 in, 2 out]
                n194 = Reciprocal(x=w505) -> (1/x=w484:dbl)
                n195 = local write "intercept"(w498) -> ()
                n196 = local write "residue"(w483) -> ()
                n197 = local write "Res. (ohm)"(w484) -> ()
              }
              frame #2 {
                n198 = property on="Qrun" class="Bool (strict)"("Val(Sgnl)"=FALSE ("Qrun")) -> ()  [unwired: 2 in, 2 out]
              }
            }
          }
        }
      }
      event "Reset": Value Change {
        n199 = event-data() -> ("NewVal"=w522:bool)  [unwired: 1 in]
        n200 = case shown="True" w522 {
          tunnel: [w525 w526] -> w520
          tunnel: w521 -> [w525 _]
          tunnel: w519 -> [w524 w530]
          tunnel: [w524 w529] -> w518
          tunnel: [w523 w527] -> w517
          tunnel: w516 -> [w523 w528]
          frame False {
          }
          frame True {
            n201 = call "Ke24xx Reset.vi"("error in (no error)"=w528, "instrument handle"=w530) -> ("error out"=w527:errorcluster, "status"=w526:i32, "instrument handle out"=w529:refnum<visa-resource-name>)  [unwired: 7 in]
          }
        }
      }
      event "clear graph": Value Change {
        n202 = event-data() -> ("NewVal"=w539:bool)  [unwired: 1 in]
        n203 = case shown="True" w539 {
          frame False {
          }
          frame True {
            n204 = property on="Waveform Chart" class="WFChart (strict)"("History Data"=T4 []) -> ()  [unwired: 2 in, 2 out]
          }
        }
      }
    }
    "status" <- w65
    "KEITHLEY error IO" <- w60
    "DAQ error IO" <- w52
    n205 = Wait Until Next ms Multiple(millisecond multiple=u32 100) -> ()  [unwired: 1 out]
    n206 = case shown="True" "Disable MFC" {
      tunnel: w56 -> [w76 _]
      tunnel: [w75 errorcluster {"status"=TRUE, "code"=1, "source"="Disabled"} ("error out")] -> w55
      tunnel: w54 -> [w74 w85]
      tunnel: [w73 w85] -> w53
      frame False {
        n207 = case shown="Error" w76 {
          selector: w76 -> [w78 w81]
          tunnel: [w78 w79] -> w75
          tunnel: w74 -> [w77 w83]
          tunnel: [w77 w82] -> w73
          frame No Error {
          }
          frame Error {
            n208 = VISA Clear(VISA resource name=w83, error in (no error)=w81) -> (VISA resource name out=w82:refnum<visa-resource-name>, error out=w80:errorcluster)
            n209 = call <vilib>:"Clear Errors.vi"("error in (no error)"=w80) -> ("error out"=w79:errorcluster)  [unwired: 5 in, 1 out]
          }
        }
      }
      frame True {
      }
    }
    "MFC error IO" <- w55
  }
  n210 = call "Ke24xx Close.vi"("error in (no error)"=w43, "instrument handle"=w44) -> ("error out"=w25:errorcluster)  [unwired: 8 in, 1 out]
  n211 = call <vilib>:"DAQmx Stop Task.vi"("task/channels in"=w9, "error in"=w8) -> ("task out"=w11:refnum<k21>, "error out"=w10:errorcluster)  [unwired: 12 in]
  n212 = call <vilib>:"DAQmx Clear Task.vi"("task in"=w11, "error in"=w10) -> ("error out"=w7:errorcluster)  [unwired: 13 in]
  n213 = call <vilib>:"Clear Errors.vi"("error in (no error)"=w25) -> ()  [unwired: 5 in, 2 out]
  n214 = VISA Close(VISA resource name=w28, error in (no error)=w27) -> (error out=w26:errorcluster)
  n215 = call <vilib>:"Clear Errors.vi"("error in (no error)"=w7) -> ()  [unwired: 5 in, 2 out]
  n216 = call <vilib>:"Clear Errors.vi"("error in (no error)"=w26) -> ()  [unwired: 5 in, 2 out]
